vi "10 Add.vi"() -> ()   [LabVIEW 2018]
panel:
  out "C":dbl
  in  "B":dbl
  in  "A":dbl
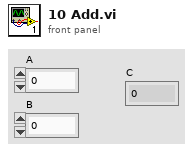
[diagram p1: front panel]
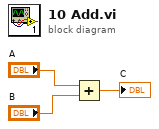
[diagram p0: block diagram]
diagram:
  n1 = Add(x="A", y="B") -> (x+y=→"C":dbl)
